vi "Waveform Generator [Express].vi"() -> ()   [LabVIEW 2017]
panel:
  out "error out":errorcluster
  in  "Digitizing Parameters":T1={"Numbers of Samples"=100, "Sampling Frequency"=1000.0}
  in  "Waveform Parameters":T2={"Frequency"=50.0, "Amplitude"=5.0, "Shape"=enum."Sine"}
  out "XY Graph":cluster{"Displacement":dbl[], "Time":dbl[]}(graph)
  in  "stop":bool
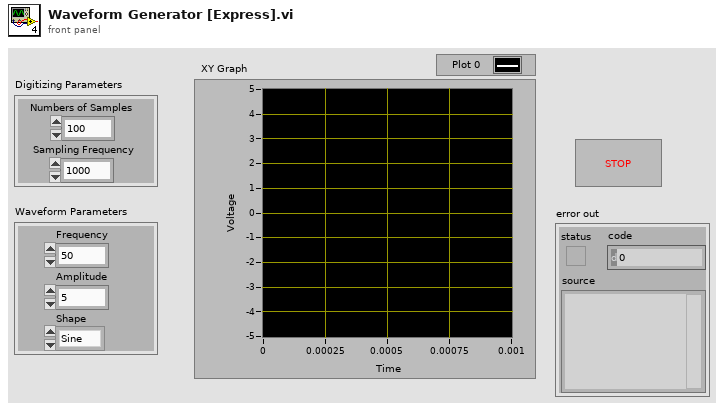
[diagram p1: front panel]
types:
  T1 = cluster{"Numbers of Samples":i32, "Sampling Frequency":dbl}
  T2 = cluster{"Frequency":dbl, "Amplitude":dbl, "Shape":enum16{"Sine", "Cosine", "DC Level", "Square", "User-Defined"}}
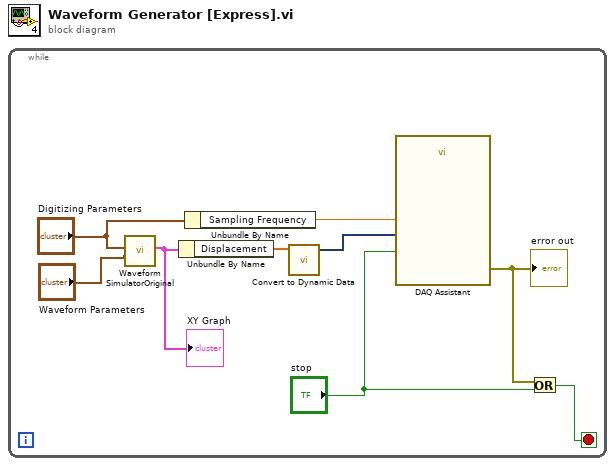
[diagram p0: block diagram]
diagram:
  n1 = while {
    stop <- w4 stop-if-true
    n2 = call "Waveform SimulatorOriginal.vi"("Waveform Parameters"="Waveform Parameters", "Digitizing Parameters"="Digitizing Parameters") -> ("Waveform Output"=w1:cluster{"Time":dbl[], "Displacement":dbl[]})  [unwired: 9 in]
    "XY Graph" <- w1
    n3 = Unbundle By Name(w1) -> ("Displacement"=w8:dbl[])
    n4 = Unbundle By Name("Digitizing Parameters") -> ("Sampling Frequency"=w9:dbl)
    n5 = call "Convert to Dynamic Data"("Array"=w8) -> ("Dynamic Data Type"=w7:dynamicdata)  [unwired: 3 in]
    n6 = call "DAQ Assistant"("data"=w7, "rate"=w9, "stop (F)"="stop") -> ("error out"=w6:errorcluster)  [unwired: 14 in, 2 out]
    "error out" <- w6
    n7 = Or(x=w6, y="stop") -> (x .or. y?=w4:bool)
  }
